vi "LVClass_WavefrontCorrectorSet Get Parameter String List One Element.vi"(0 "WavefrontCorrectorSet in":refnum<class "WavefrontCorrectorSet.lvclass">, 5 "parameter name":string, 7 "index":u32, 11 "error in (no error)":errorcluster) -> (4 "WavefrontCorrectorSet out":refnum<class "WavefrontCorrectorSet.lvclass">, 6 "value":string, 15 "error out":errorcluster)   [LabVIEW 2020, in "WavefrontCorrectorSet.lvclass"]
doc: "If parameter is a string to be selected among a finite set of strings,\nextract the possible value located at the /p index position from this set.\nSee Imop_WavefrontCorrectorSet_GetParameterOption.\n\n--------------------------------------------------------------------------------\n\n<B>wavefrontcorrector_setIn </B> : WavefrontCorrectorSet object.\n<B>wavefrontcorrector_setOut </B> : WavefrontCorrectorSet object.\n<B>parameter_name </B> : Parameter name (must be the name of a parameter of type strings list).\n<B>index </B> : Sub-parameter index.\n<B>value </B> : Value at index index.\n<B>ErrorIn </B> : Error\n<B>ErrorOut </B> : Error\n\n--------------------------------------------------------------------------------"
uses:
  WavefrontCorrectorSet.lvclass
  WavefrontCorrectorSet.lvclass/WavefrontCorrectorSet.ctl
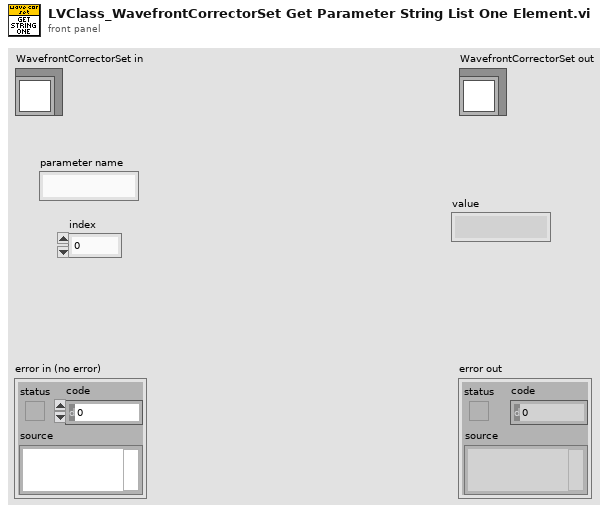
[diagram p1: front panel]
types:
  T1 = typedef "ClassID.ctl" = i64
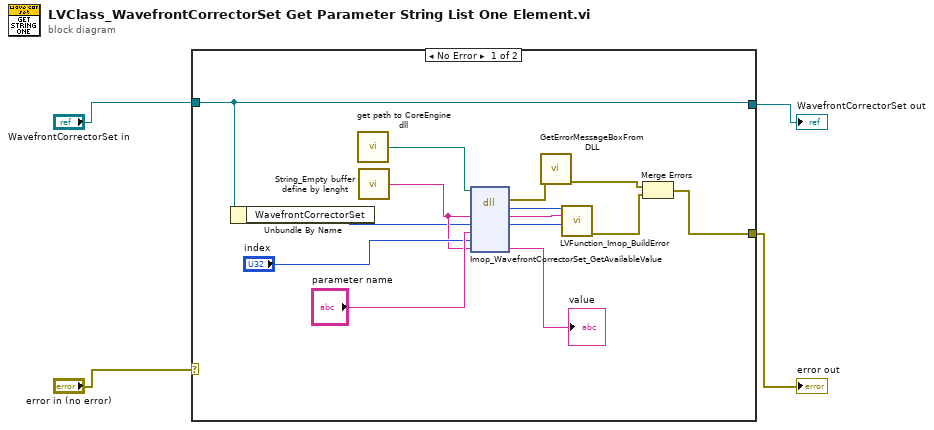
[diagram p0: block diagram]
diagram:
  n1 = case shown="No Error" "error in (no error)" {
    selector: "error in (no error)" -> [_ w19]
    tunnel: "WavefrontCorrectorSet in" -> [w10 w20]
    tunnel: [w10 w20] -> w1
    tunnel: [w6 w19] -> w2
    frame No Error {
      n2 = Unbundle By Name(w10) -> ("WavefrontCorrectorSet"=w9:T1)
      n3 = call "get path to CoreEngine dll.vi"() -> ("path to wavekit library"=w15:path)  [unwired: 14 in, 1 out]
      n4 = call "String_Empty buffer define by lenght.vi"() -> ("Empty buffer"=w12:string)  [unwired: 1 in]
      n5 = dll-call lib="D:/soft/HASO_v3/SVN_trunk/ImOpCoreEngine4_LV2011/DLLs/c_interface_vc100.dll" fn="Imop_WavefrontCorrectorSet_GetAvailableValue"(path in=w15, "message"=w12, "objet"=w9, "parameter name"="parameter name", "index"="index", "Name"=w12) -> (error out=w14:errorcluster, "return type"=w18:i32, "message"=w17:string, "objet"=w5:i64, "Name"=→"value":string)  [unwired: 4 in, 1 out]
      n6 = call "GetErrorMessageBoxFromDLL.vi"("error IN"=w14) -> ("error OUT"=w8:errorcluster)  [unwired: 10 in]
      n7 = call "LVFunction_Imop_BuildError.vi"("code"=w18, "String to Prepend to source (\"\")"=w17, "Adresse"=w5) -> ("error out"=w7:errorcluster)  [unwired: 12 in]
      n8 = Merge Errors(w8, w7) -> (w6:errorcluster)
    }
    frame Error {
    }
  }
  "error out" <- w2
  "WavefrontCorrectorSet out" <- w1
